vi "Path Is Filled.vi"(8 "error in (no error)":errorcluster, 11 "Tool Path in":refnum<class "Tool Path.lvclass">) -> (0 "error out":errorcluster, 2 "Filled?":bool, 3 "Tool Path out":refnum<class "Tool Path.lvclass">)   [LabVIEW 2019, in "Tool Path.lvclass"]
uses:
  Tool Path.lvclass
  Parse/CSSProperties/CSSProperties.lvclass
  Parse/ParsePaths/Path.lvclass
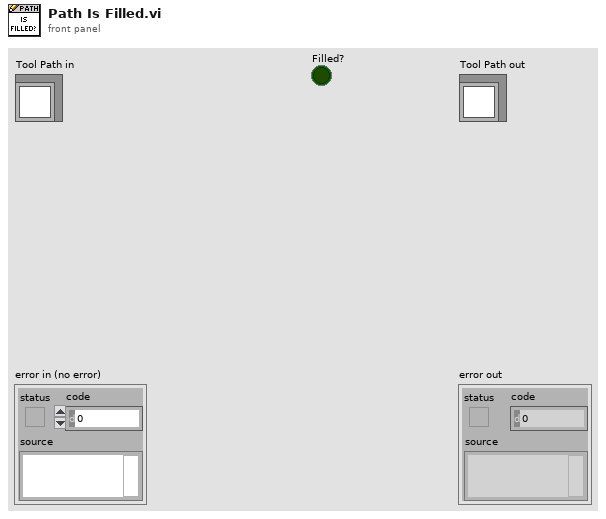
[diagram p1: front panel]
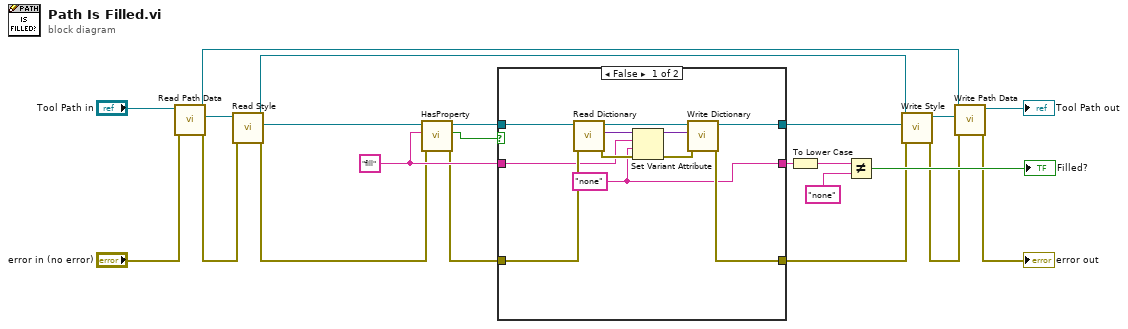
[diagram p0: block diagram]
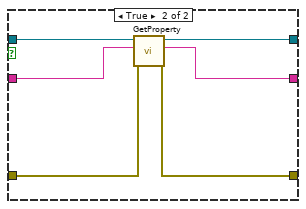
[diagram p2: hidden frame]
diagram:
  w21 = "fill" ("Property")
  n1 = call-dynamic "Read Path Data.vi"("error in (no error)"="error in (no error)", "Tool Path in"="Tool Path in") -> ("error out"=w11:errorcluster, "Path.lvclass"=w15:refnum<class "Path.lvclass">, "Tool Path out"=w2:refnum<class "Tool Path.lvclass">)  [unwired: 7 in]
  n2 = call "Read Style.vi"("error in (no error)"=w11, "Path in"=w15) -> ("error out"=w10:errorcluster, "CSSProperties.lvclass"=w14:refnum<class "CSSProperties.lvclass">, "Path out"=w1:refnum<class "Path.lvclass">)  [unwired: 7 in]
  n3 = call "HasProperty.vi"("error in (no error)"=w10, "Property"=w21, "CSSProperties in"=w14) -> ("error out"=w13:errorcluster, "Exists?"=w22:bool, "CSSProperties out"=w20:refnum<class "CSSProperties.lvclass">)  [unwired: 6 in]
  n4 = case shown="False" w22 {
    tunnel: [w30 w39] -> w9
    tunnel: [w23 w35] -> w19
    tunnel: w20 -> [w29 w38]
    tunnel: w21 -> [w24 w34]
    tunnel: [w28 w37] -> w5
    tunnel: w13 -> [w27 w36]
    frame False {
      w23 = "none" ("Value")
      n5 = call "Read Dictionary.vi"("error in (no error)"=w27, "CSSProperties in"=w29) -> ("error out"=w25:errorcluster, "Dictionary"=w32:variant, "CSSProperties out"=w31:refnum<class "CSSProperties.lvclass">)  [unwired: 7 in]
      n6 = Set Variant Attribute(Variant=w32, name=w24, value=w23, error in=w25) -> (Variant out=w33:variant, error out=w26:errorcluster)  [unwired: 1 out]
      n7 = call "Write Dictionary.vi"("error in (no error)"=w26, "Dictionary"=w33, "CSSProperties in"=w31) -> ("error out"=w28:errorcluster, "CSSProperties out"=w30:refnum<class "CSSProperties.lvclass">)  [unwired: 7 in]
    }
    frame True {
      n8 = call "GetProperty.vi"("error in (no error)"=w36, "Property"=w34, "CSSProperties in"=w38) -> ("error out"=w37:errorcluster, "Value"=w35:string, "CSSProperties out"=w39:refnum<class "CSSProperties.lvclass">)  [unwired: 6 in]
    }
  }
  n9 = To Lower Case(string=w19) -> (all lower case string=w18:string)
  n10 = Not Equal?(x=w18, y="none") -> (x != y?=→"Filled?":bool)
  n11 = call "Write Style.vi"("error in (no error)"=w5, "CSSProperties.lvclass"=w9, "Path in"=w1) -> ("error out"=w3:errorcluster, "Path out"=w8:refnum<class "Path.lvclass">)  [unwired: 7 in]
  n12 = call-dynamic "Write Path Data.vi"("error in (no error)"=w3, "Path.lvclass"=w8, "Tool Path in"=w2) -> ("error out"=→"error out":errorcluster, "Tool Path out"=→"Tool Path out":refnum<class "Tool Path.lvclass">)  [unwired: 7 in]
